vi "Network Steam Connect.vi"(6 "Timeout(ms)":i32=500, 8 "error in (no error)":errorcluster, 11 "Model_AMC in":refnum<class "Model_AMC.lvclass">) -> (0 "error out":errorcluster, 2 "Connected?":bool, 3 "Model_AMC out":refnum<class "Model_AMC.lvclass">)   [LabVIEW 2021, in "Model_AMC.lvclass"]
uses:
  Model_AMC.lvclass
  Model_AMC.lvclass/Model_AMC.ctl
  <userlib>/John_Lib/Network_Streams_Connection/NetworkConnection.lvclass
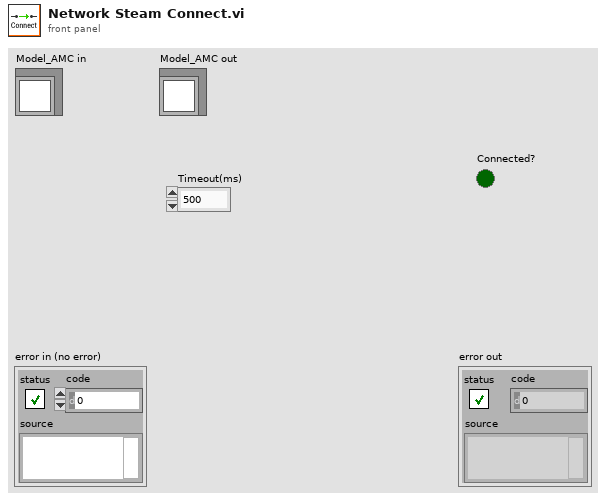
[diagram p1: front panel]
types:
  T1 = typedef "Model_AMC.lvclass/DVR.ctl" = cluster{"JKI_Network_Streams":refnum<class "NetworkConnection.lvclass">, "AMC Q":T2}
  T2 = typedef "Model_AMC.lvclass/AMC Q.ctl" = cluster{"Main":T3, "OPCUA":T3, "NetworkSteam":T3}
  T3 = typedef "AMC_FW.lvlib/Queue.ctl" = cluster{"Q":T4, "Name":string}
  T4 = typedef "AMC_FW.lvlib/Message Queue.ctl" = refnum<queue>
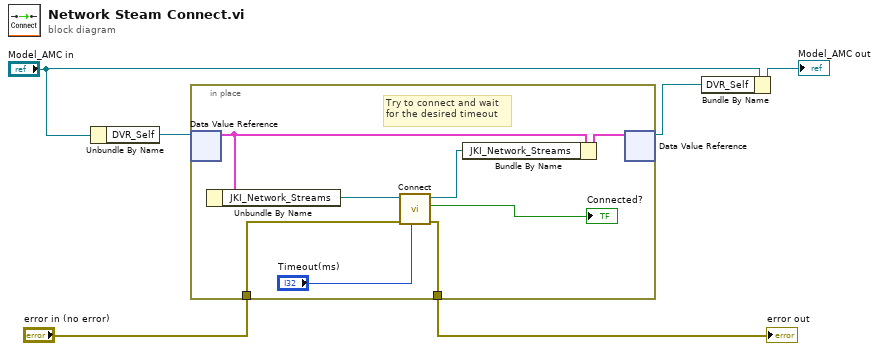
[diagram p0: block diagram]
diagram:
  n1 = Unbundle By Name("Model_AMC in") -> ("DVR_Self"=w6:refnum<data-value>)
  n2 = in-place {
    in-place-border: [w8] -> w5
    in-place-border: "error in (no error)" -> [w7]
    # "Try to connect and wait\nfor the desired timeout"
    n3 = in-place-dvr #1(w6) -> (w13:T1)  [unwired: 1 out]
    n4 = Unbundle By Name(w13) -> ("JKI_Network_Streams"=w12:refnum<class "NetworkConnection.lvclass">)
    n5 = call <userlib>:"Connect.vi"("Timeout(ms)"="Timeout(ms)", "error in (no error)"=w7, "NetworkConnection in"=w12) -> ("error out"=w8:errorcluster, "Connected?"=→"Connected?":bool, "NetworkConnection out"=w10:refnum<class "NetworkConnection.lvclass">)  [unwired: 6 in]
    n6 = Bundle By Name(cluster=w13, "JKI_Network_Streams"=w10) -> (w11:T1)
    n7 = in-place-dvr #1(w11) -> (w1:refnum<data-value>)  [unwired: 1 out]
  }
  "error out" <- w5
  n8 = Bundle By Name(cluster="Model_AMC in", "DVR_Self"=w1) -> (→"Model_AMC out":refnum<class "Model_AMC.lvclass">)
